vi "FaultGetValue.vi"(9 "Channel":string, 11 "ChannelFault in":T1) -> (0 "error out":errorcluster, 1 "Channel out":string, 2 "Faulted":bool, 3 "Fault Value":dbl)   [LabVIEW 2015, in "MiscHelperVIs.lvlib"]
uses:
  MiscHelperVIs.lvlib
  <vilib>/NI Veristand/Execution/ChannelFaultManager/ChannelFaultAPI.ctl
  NationalInstruments.VeriStand.ClientAPI
  <vilib>/NI Veristand/Execution/ChannelFaultManager/NI_VS ChannelFault ExecutionAPI.lvlib
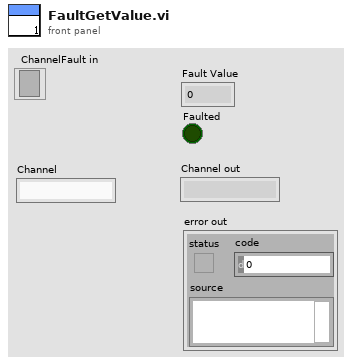
[diagram p1: front panel]
types:
  T1 = typedef "NI_VS ChannelFault ExecutionAPI.lvlib/ChannelFaultAPI.ctl" = refnum<k24>
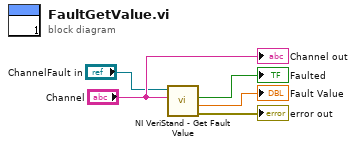
[diagram p0: block diagram]
diagram:
  n1 = call <vilib>:"NI VeriStand - Get Fault Value.vi"("Channel"="Channel", "ChannelFault in"="ChannelFault in") -> ("error out"=→"error out":errorcluster, "Fault Value"=→"Fault Value":dbl, "Faulted"=→"Faulted":bool)  [unwired: 6 in, 1 out]
  "Channel out" <- "Channel"
